vi "SteeringControlSimulation.vi"() -> ()   [LabVIEW 2016]
uses:
  <vilib>/rvi/Analysis/control/PID/Typedef/niFpgaPID_PIDActions.ctl
  <vilib>/rvi/Analysis/control/PID/Typedef/niFpgaPID_SetpointWeightings.ctl
  <vilib>/rvi/Analysis/control/PID/Typedef/niFpgaPID_OutputRange.ctl
  <vilib>/rvi/Analysis/control/PID/Typedef/niFpgaPID_PIDGains.ctl
  <vilib>/rvi/Emulation/niFpgaGetClockAttributes.vi
  <vilib>/rvi/Emulation/niFpgaSctlEmulationGetInTimedLoop.vi
  <vilib>/rvi/Emulation/niFpgaEmulationReportErrorSimple.vi
  <vilib>/rvi/Analysis/control/PID/SubVIs/niFpgaPID_PIDWrapper.vi
  <vilib>/rvi/Emulation/niFpgaCriticalErrorInLSC.vi
panel:
  in  "Direction":bool
  out "Position":i64
  in  "Desired steering angle":sgl format="%#_13g"
  in  "gains":T1 {"filter coefficient" min=0 max=1; "proportional gain" step=0.125}
  in  "output range":T2={"output high (Inf)"=inf, "output low (-Inf)"=-inf}
  in  "setpoint weighting":T3={"proportional weighting (1)"=1.0, "derivative weighting (0)"=0.0} {"derivative weighting (0)" min=0 max=1; "proportional weighting (1)" min=0 max=1}
  out "Setpoint error":sgl
  out "accual PID values":T4
  in  "Stop PID controller":bool
  in  "Pid reset (F)":bool
  out "Duty cycle (steering)":sgl
  in  "Current steering angle":sgl
  out "Steering loop time":u32
  in  "loop wait time (ticks)":u32 caption="Count(mSec)"
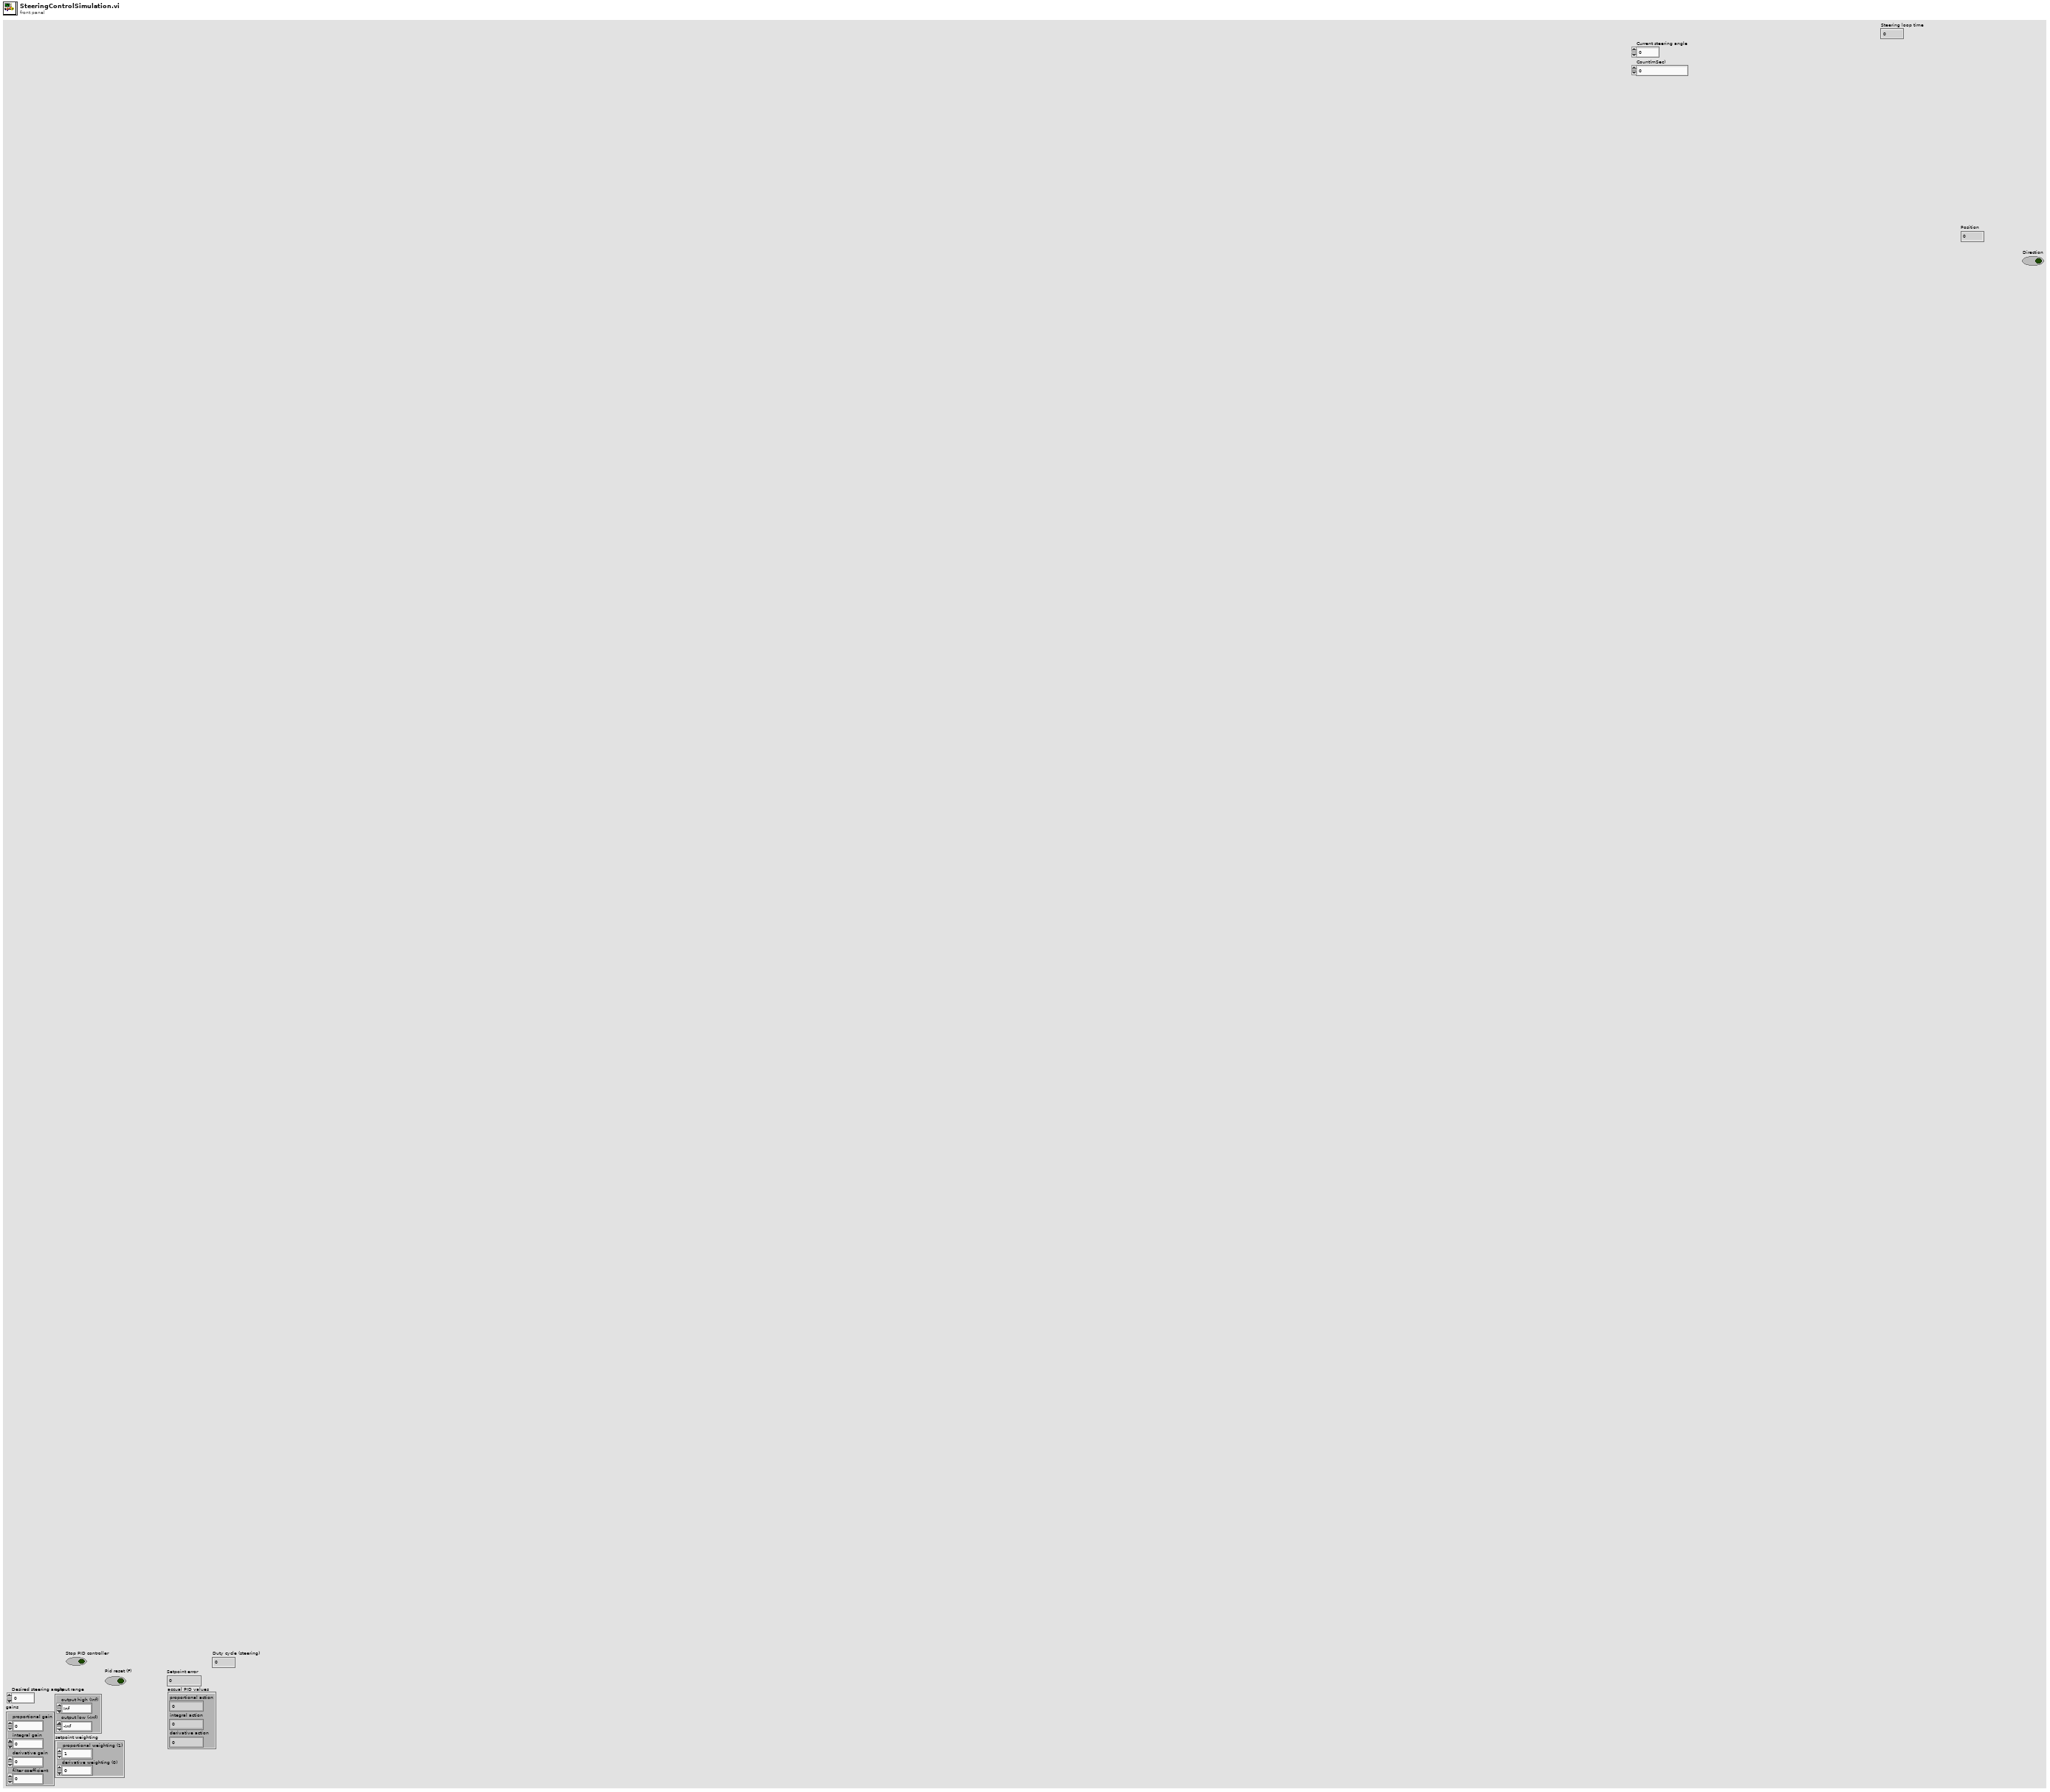
[diagram p1: front panel]
types:
  T1 = typedef "niFpgaPID_PIDGains.ctl" = cluster{"proportional gain":sgl, "integral gain":sgl, "derivative gain":sgl, "filter coefficient":sgl}
  T2 = typedef "niFpgaPID_OutputRange.ctl" = cluster{"output high (Inf)":sgl, "output low (-Inf)":sgl}
  T3 = typedef "niFpgaPID_SetpointWeightings.ctl" = cluster{"proportional weighting (1)":sgl, "derivative weighting (0)":sgl}
  T4 = typedef "niFpgaPID_PIDActions.ctl" = cluster{"proportional action":sgl, "integral action":sgl, "derivative action":sgl}
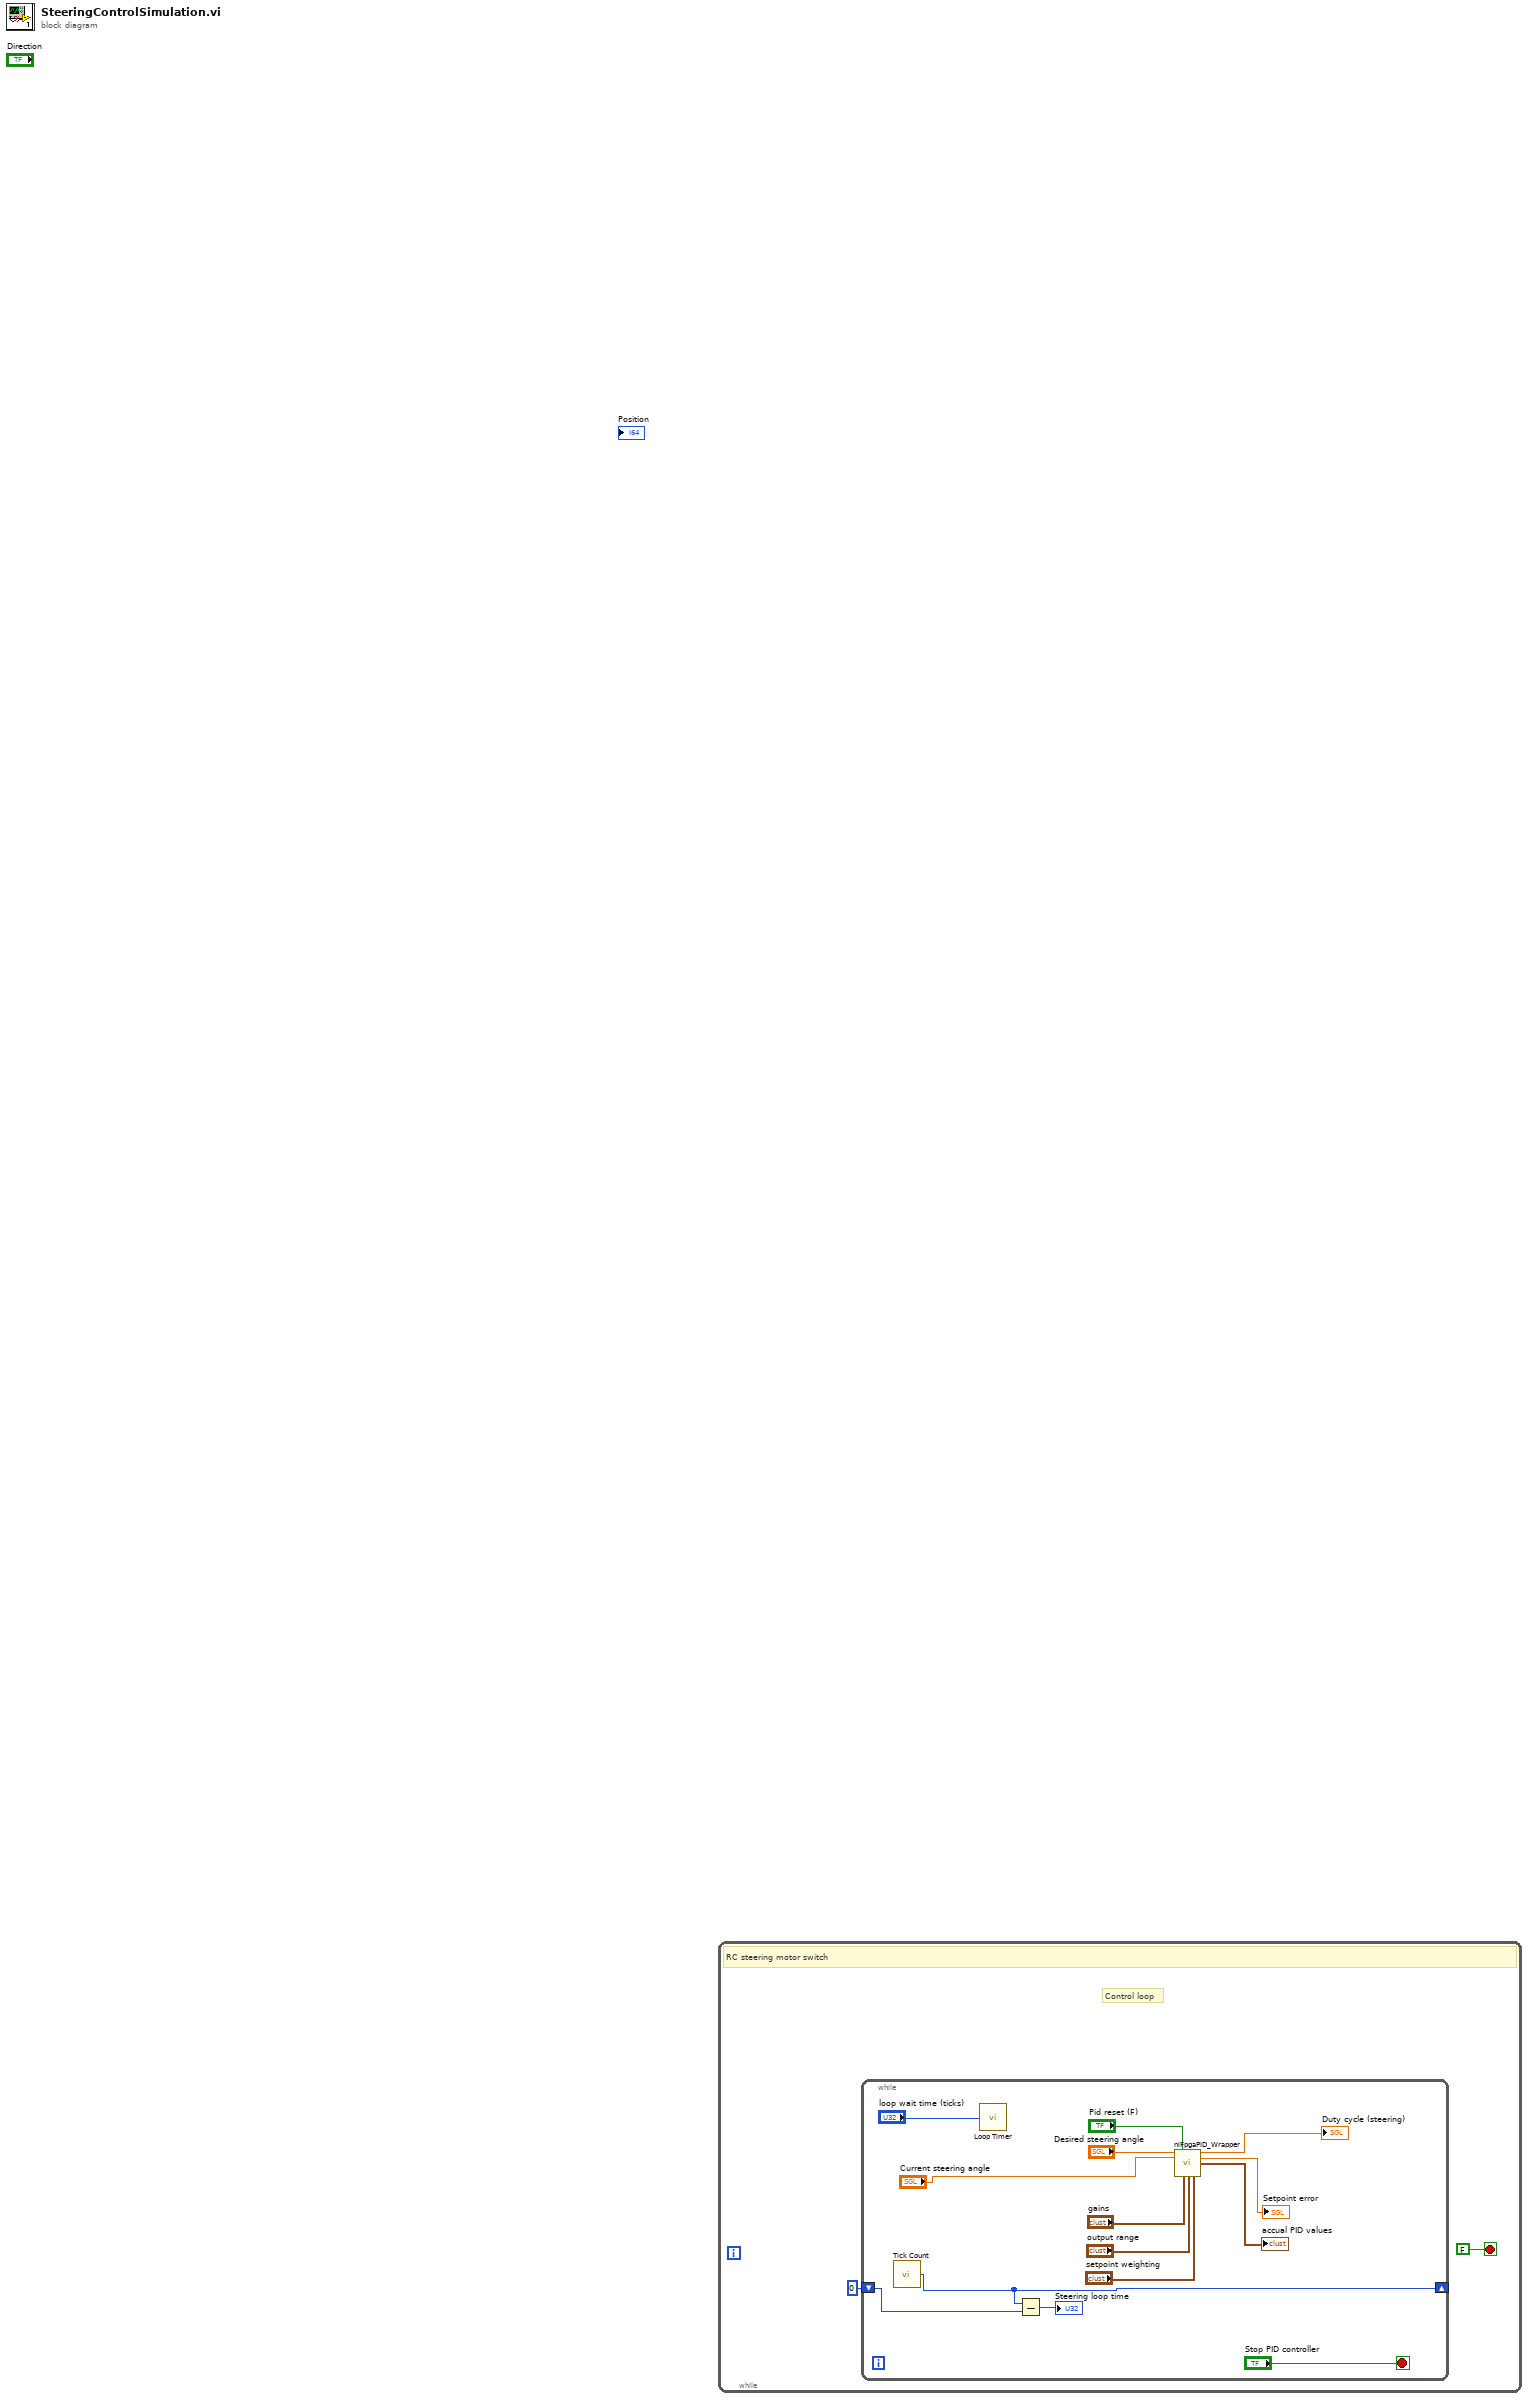
[diagram p0: block diagram]
diagram:
  n1 = while {
    stop <- FALSE stop-if-true
    # "Control loop"
    # "RC steering motor switch"
    n2 = while {
      shift-right: [w8] -> _
      shift-left: u32 0 ("Tick Count(Ticks)") -> [w9]
      stop <- "Stop PID controller" stop-if-true
      n3 = call "Tick Count"() -> ("Tick Count(Ticks)"=w8:u32)
      n4 = call "Loop Timer"("Count(Ticks)"="loop wait time (ticks)") -> ()  [unwired: 1 out]
      n5 = Subtract(x=w8, y=w9) -> (x-y=→"Steering loop time":u32)
      n6 = call-poly <vilib>:"niFpgaPID_Wrapper.vi"("setpoint"="Desired steering angle", "reset? (F)"="Pid reset (F)", "process variable"="Current steering angle", "gains"="gains", "output range"="output range", "setpoint weighting"="setpoint weighting") -> ("output"=→"Duty cycle (steering)":sgl, "error"=→"Setpoint error":sgl, "actions"=→"accual PID values":T4)  [unwired: 7 in]
    }
  }
